vi "start.vi"(8 "error in":errorcluster, 10 "start":bool=TRUE, 11 "profibus reference":T1) -> (0 "error out":errorcluster, 3 "profibus reference out":T1)   [LabVIEW 2013, in "dynamic profibus.lvlib"]
uses:
  dynamic profibus.lvlib
  fpga reference.ctl
  <vilib>/rvi/interface/common/niFpgaWaitOnOcc.vi
  <vilib>/Utility/error.llb/Error Cluster From Error Code.vi
  <vilib>/rvi/errors/niLvFpgaAdjustHostInterfaceError.vi
  <vilib>/rvi/interface/nirviReadWriteControl/nirviReadWriteControl.xnode
  NiFpgaLv.dll
  <vilib>/rvi/interface/Simulation/niFpgaSimulationCallBeginRW.vi
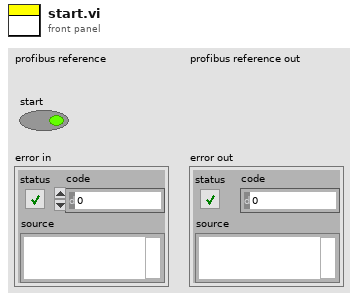
[diagram p1: front panel]
types:
  T1 = typedef "dynamic profibus.lvlib/fpga reference.ctl" = refnum<k20>
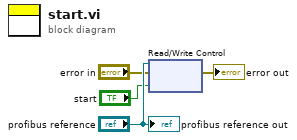
[diagram p0: block diagram]
diagram:
  n1 = xnode "Read/Write Control"("FPGA VI Reference In"="profibus reference", "error in"="error in", "start"="start") -> ("error out"=→"error out":errorcluster)  [unwired: 1 out]
  "profibus reference out" <- "profibus reference"
